vi "Find.vi"(8 "error in":errorcluster, 11 "target in":refnum<k24>) -> (0 "error out":errorcluster, 2 "Ballard ARINC 429 custom devices":u64[](array[numeric]) format="%.0x", 3 "target out":refnum<k24>)   [LabVIEW 2020, in "Ballard ARINC 429 Scripting.lvlib"]
uses:
  Ballard ARINC 429 Scripting.lvlib
  NationalInstruments.VeriStand.SystemDefinitionAPI
  Constants.vi
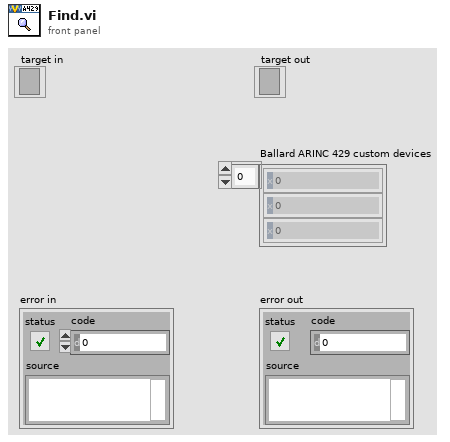
[diagram p1: front panel]
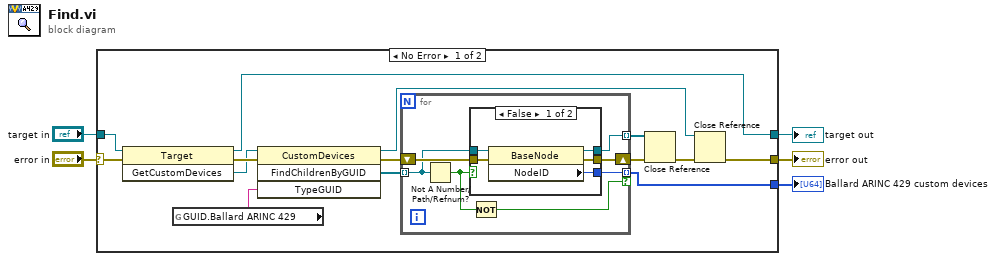
[diagram p0: block diagram]
diagram:
  n1 = case shown="No Error" "error in" {
    selector: "error in" -> [w13 w35]
    tunnel: "target in" -> [w15 w34]
    tunnel: [w8 w35] -> w3
    tunnel: [w7 _] -> w1
    tunnel: [w10 w34] -> w2
    frame No Error {
      n2 = invoke class="Target" method="GetCustomDevices"(reference=w15, error in=w13) -> (reference out=w10:refnum<k24>, error out=w19:errorcluster, "GetCustomDevices"=w18:refnum<k24>)  [unwired: 1 in]
      n3 = global read "Constants.vi" "GUID.Ballard ARINC 429"() -> (w6:string)
      n4 = invoke class="CustomDevices" method="FindChildrenByGUID"(reference=w18, error in=w19, "TypeGUID"=w6) -> (reference out=w11:refnum<k24>, error out=w9:errorcluster, "FindChildrenByGUID"=w14:refnum<k24>[])  [unwired: 1 in, 1 out]
      n5 = for {
        shift-right: [w24] -> w16
        shift-left: w9 -> [w26]
        tunnel: w14 -> [w23] mode=indexing
        tunnel: [w25] -> w17 mode=indexing
        tunnel: [w22] -> w7 mode=indexing if=w20
        n6 = Not A Number/Path/Refnum?(number/path/refnum=w23) -> (NaN/Path/Refnum?=w21:bool)
        n7 = case shown="False" w21 {
          tunnel: [w28 w33] -> w24
          tunnel: w26 -> [w30 w33]
          tunnel: w23 -> [w31 w32]
          tunnel: [w29 w32] -> w25
          tunnel: [w27 _] -> w22
          frame False {
            n8 = property class="BaseNode"(reference=w31, error in=w30) -> (reference out=w29:refnum<k24>, error out=w28:errorcluster, "NodeID"=w27:u64)
          }
          frame True {
          }
        }
        n9 = Not(x=w21) -> (.not. x?=w20:bool)
      }
      n10 = Close Reference(reference=w17, error in (no error)=w16) -> (error out=w12:errorcluster)
      n11 = Close Reference(reference=w11, error in (no error)=w12) -> (error out=w8:errorcluster)
    }
    frame Error {
    }
  }
  "error out" <- w3
  "target out" <- w2
  "Ballard ARINC 429 custom devices" <- w1
